vi "Configure Trigger (Edge).vi"(0 "VISA resource name":refnum<visa-resource-name>, 1 "Trigger Coupling (1 : DC)":u16(ring)=1 items=["AC", "DC", "Low Freq Reject", "High Freq Reject"], 5 "Trigger Source (1: Channel 1)":i32(ring)=1 items=["Channel 1"=1, "Channel 2"=2, "Channel 3"=3, "Channel 4"=4, "Digital 0"=13, "Digital 1"=14, "Digital 2"=15, "Digital 3"=16, "Digital 4"=17, "Digital 5"=18, "Digital 6"=19, "Digital 7"=20, "Digital 8"=21, "Digital 9"=22, "Digital 10"=23, "Digital 11"=24, "Digital 12"=25, "Digital 13"=26, "Digital 14"=27, "Digital 15"=28, "Aux"=29, "Line"=30], 7 "Trigger Level (0.0 V)":dbl, 9 "Trigger Slope (0: Positive)":u16(ring) items=["Positive", "Negative"], 11 "error in (no error)":errorcluster) -> (4 "VISA resource name out":refnum<visa-resource-name>, 15 "error out":errorcluster)   [LabVIEW 2012, in "Agilent 8000 Series.lvlib"]
doc: "Configures edge trigger settings. An edge trigger occurs when the trigger signal passes through the voltage threshold that you specify with the <B>Trigger Level</B> control and has the slope that you specify with the <B>Trigger Slope</B> control. \n\n<B>Note:</B>\nThe 80000 Series Oscilloscopes <B>do not</B> support Trigger Coupling."
uses:
  Agilent 8000 Series.lvlib
panel:
  # "80000 Series Oscilloscopes do\nnot support Trigger Coupling"
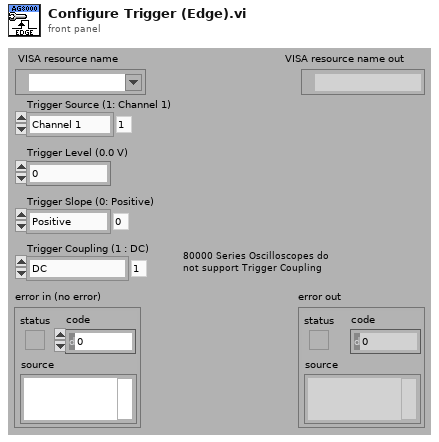
[diagram p1: front panel]
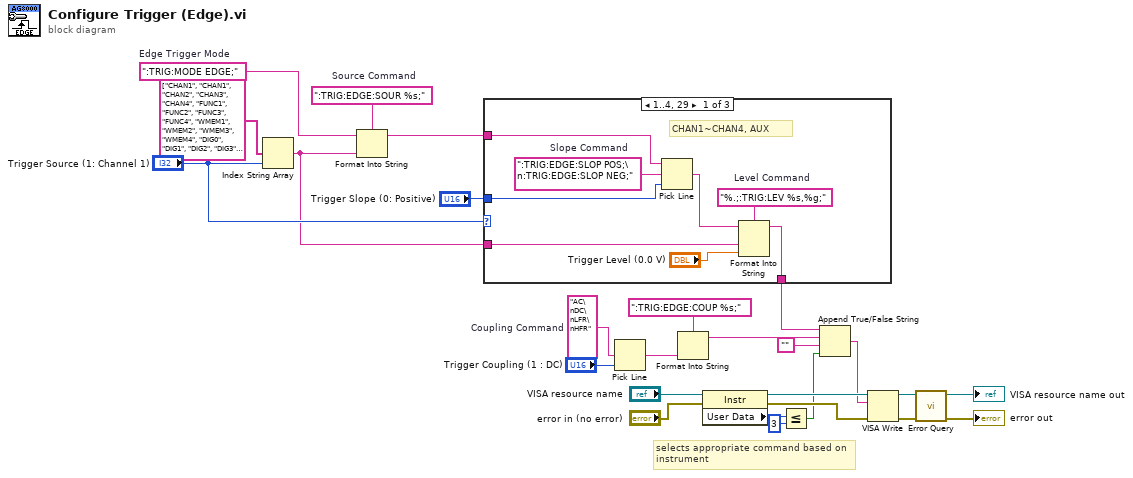
[diagram p0: block diagram]
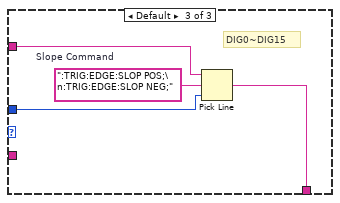
[diagram p3: hidden frame]
diagram:
  w15 = "AC\nDC\nLFR\nHFR"  # Coupling Command
  w19 = ":TRIG:MODE EDGE;"  # Edge Trigger Mode
  w22 = ":TRIG:EDGE:SOUR %s;"  # Source Command
  # "selects appropriate command based on instrument"
  n1 = Index String Array(1:"Trigger Source (1: Channel 1)", 2:string[] ["CHAN1", "CHAN1", "CHAN2", "CHAN3", "CHAN4", "FUNC1", "FUNC2", "FUNC3", "FUNC4", "WMEM1", "WMEM2", "WMEM3", "WMEM4", "DIG0", "DIG1", "DIG2", "DIG3", "DIG4", "DIG5", "DIG6", "DIG7", "DIG8", "DIG9", "DIG10", "DIG11", "DIG12", "DIG13", "DIG14", "DIG15", "AUX", "LINE"]) -> (0:w17:string)  [unwired: 1 in]
  n2 = Format Into String(format string=w22, initial string=w19, w17) -> (resulting string=w12:string)  [unwired: 1 in, 1 out]
  n3 = case shown="1..4, 29" "Trigger Source (1: Channel 1)" {
    tunnel: [w32 w35 w36] -> w5
    tunnel: "Trigger Slope (0: Positive)" -> [w29 _ w38]
    tunnel: w12 -> [w30 w35 w37]
    tunnel: w17 -> [w27 _ _]
    frame 1..4, 29 {
      w31 = ":TRIG:EDGE:SLOP POS;\n:TRIG:EDGE:SLOP NEG;"  # Slope Command
      w33 = "%.;:TRIG:LEV %s,%g;"  # Level Command
      # "CHAN1~CHAN4, AUX"
      n4 = Pick Line(string ("")=w30, multi-line string=w31, line index=w29) -> (output string=w28:string)
      n5 = Format Into String(format string=w33, initial string=w28, w27, "Trigger Level (0.0 V)") -> (resulting string=w32:string)  [unwired: 1 in, 1 out]
    }
    frame 30 {
      # "LINE"
    }
    frame Default {
      w39 = ":TRIG:EDGE:SLOP POS;\n:TRIG:EDGE:SLOP NEG;"  # Slope Command
      # "DIG0~DIG15"
      n6 = Pick Line(string ("")=w37, multi-line string=w39, line index=w38) -> (output string=w36:string)
    }
  }
  n7 = Pick Line(multi-line string=w15, line index="Trigger Coupling (1 : DC)") -> (output string=w14:string)  [unwired: 1 in]
  n8 = Format Into String(format string=":TRIG:EDGE:COUP %s;", w14) -> (resulting string=w6:string)  [unwired: 2 in, 1 out]
  n9 = property class="Instr"(reference="VISA resource name", error in="error in (no error)") -> (reference out=w9:refnum<visa-resource-name>, error out=w8:errorcluster, "User Data"=w11:u32)
  n10 = Less Or Equal?(x=w11, y=u32 3) -> (x <= y?=w4:bool)
  n11 = Append True/False String(1:w4, 2:"", 3:w6, 4:w5) -> (0:w3:string)
  n12 = VISA Write(VISA resource name=w9, write buffer=w3, error in (no error)=w8) -> (VISA resource name out=w24:refnum<visa-resource-name>, error out=w23:errorcluster)  [unwired: 1 out]
  n13 = call "Error Query.vi"("error in (no error)"=w23, "VISA resource name"=w24) -> ("error out"=→"error out":errorcluster, "VISA resource name out"=→"VISA resource name out":refnum<visa-resource-name>)  [unwired: 6 in, 2 out]
